vi "APU + Event Timing v6 single shot.vi"() -> ()   [LabVIEW 2013]
uses:
  IP Source/APU/Input.ctl
  IP Source/APU/Output.ctl
  IP Source/APU/Settings.ctl
  IP Source/ECU Event/Timing/Capture Output.ctl
  IP Source/ECU Event/Timing/Measure Settings.ctl
  IP Source/Version Token.ctl
  IP Source/ECU Event/Timing/Measure Output.ctl
  IP Source/APU/Shared Settings.ctl
  <vilib>/Platform/TimedLoop/XDataNode/timing_clust.ctl
  <vilib>/Platform/TimedLoop/XDataNode/nitl_modes.ctl
  <vilib>/Platform/TimedLoop/XDataNode/wakeup.ctl
  IP Source/ECU Event/Timing/Capture Settings.ctl
  <vilib>/rvi/Emulation/niFpgaSctlEmulationGetInTimedLoop.vi
  <vilib>/rvi/Emulation/niFpgaEmulationReportErrorSimple.vi
  <vilib>/rvi/Emulation/niFpgaGetClockAttributes.vi
  <vilib>/rvi/Emulation/niFpgaCriticalErrorInLSC.vi
  IP Source/ECU Event/Timing/Measure Events (40MHz).vi
  <vilib>/rvi/eio/common/nirviEmuTemplateMethod_errors.vi
  <vilib>/Platform/TimedLoop/XDataNode/XDataNode.xnode
  <vilib>/eio/EIONode/EIONode.xnode
  <vilib>/Platform/TimedLoop/XDataNode/XDNodeRunTimeDep.lvlib
  IP Source/ECU Event/Timing/ECU Event Timing.lvlib
  IP Source/APU/APU.lvlib
  IP Source/Engine Simulation Toolkit.lvlib
panel:
  in  "shared settings.my apu":T1 {"cycle start" format="%#.15g"}
  in  "go.my apu":bool
  out "measure output.fi 6":T2
  out "measure output.fi 5":T2
  out "measure output.fi 4":T2
  out "measure output.fi 3":T2
  out "measure output.fi 2":T2
  out "measure output.fi 1":T2
  out "measure output.spark 6":T2
  out "measure output.spark 5":T2
  out "measure output.spark 4":T2
  out "measure output.spark 3":T2
  out "measure output.spark 2":T2
  out "measure output.spark 1":T2
  in  "est.version":T3
  out "Output.fi 1 shot 1":T4
  out "Output.fi 2 shot 1":T4
  out "Output.fi 3 shot 1":T4
  out "Output.fi 4 shot 1":T4
  out "Output.fi 5 shot 1":T4
  out "Output.fi 6 shot 1":T4
  in  "Settings.fi 1":T5
  in  "Settings.fi 2":T5
  in  "Settings.fi 3":T5
  in  "Settings.fi 4":T5
  in  "Settings.fi 5":T5
  in  "Settings.fi 6":T5
  in  "Settings.spark 6":T5
  in  "Settings.spark 5":T5
  in  "Settings.spark 4":T5
  in  "Settings.spark 3":T5
  in  "Settings.spark 2":T5
  in  "Settings.spark 1":T5
  out "Output.spark 1 shot 1":T4
  out "Output.spark 2 shot 1":T4
  out "Output.spark 3 shot 1":T4
  out "Output.spark 4 shot 1":T4
  out "Output.spark 5 shot 1":T4
  out "Output.spark 6 shot 1":T4
  in  "Settings.my apu":T6 caption="settings"
  out "Output.my apu":T7 caption="output"
  in  "Input.my apu":T8={"desired speed"=0.0, "reset"=TRUE} caption="input"
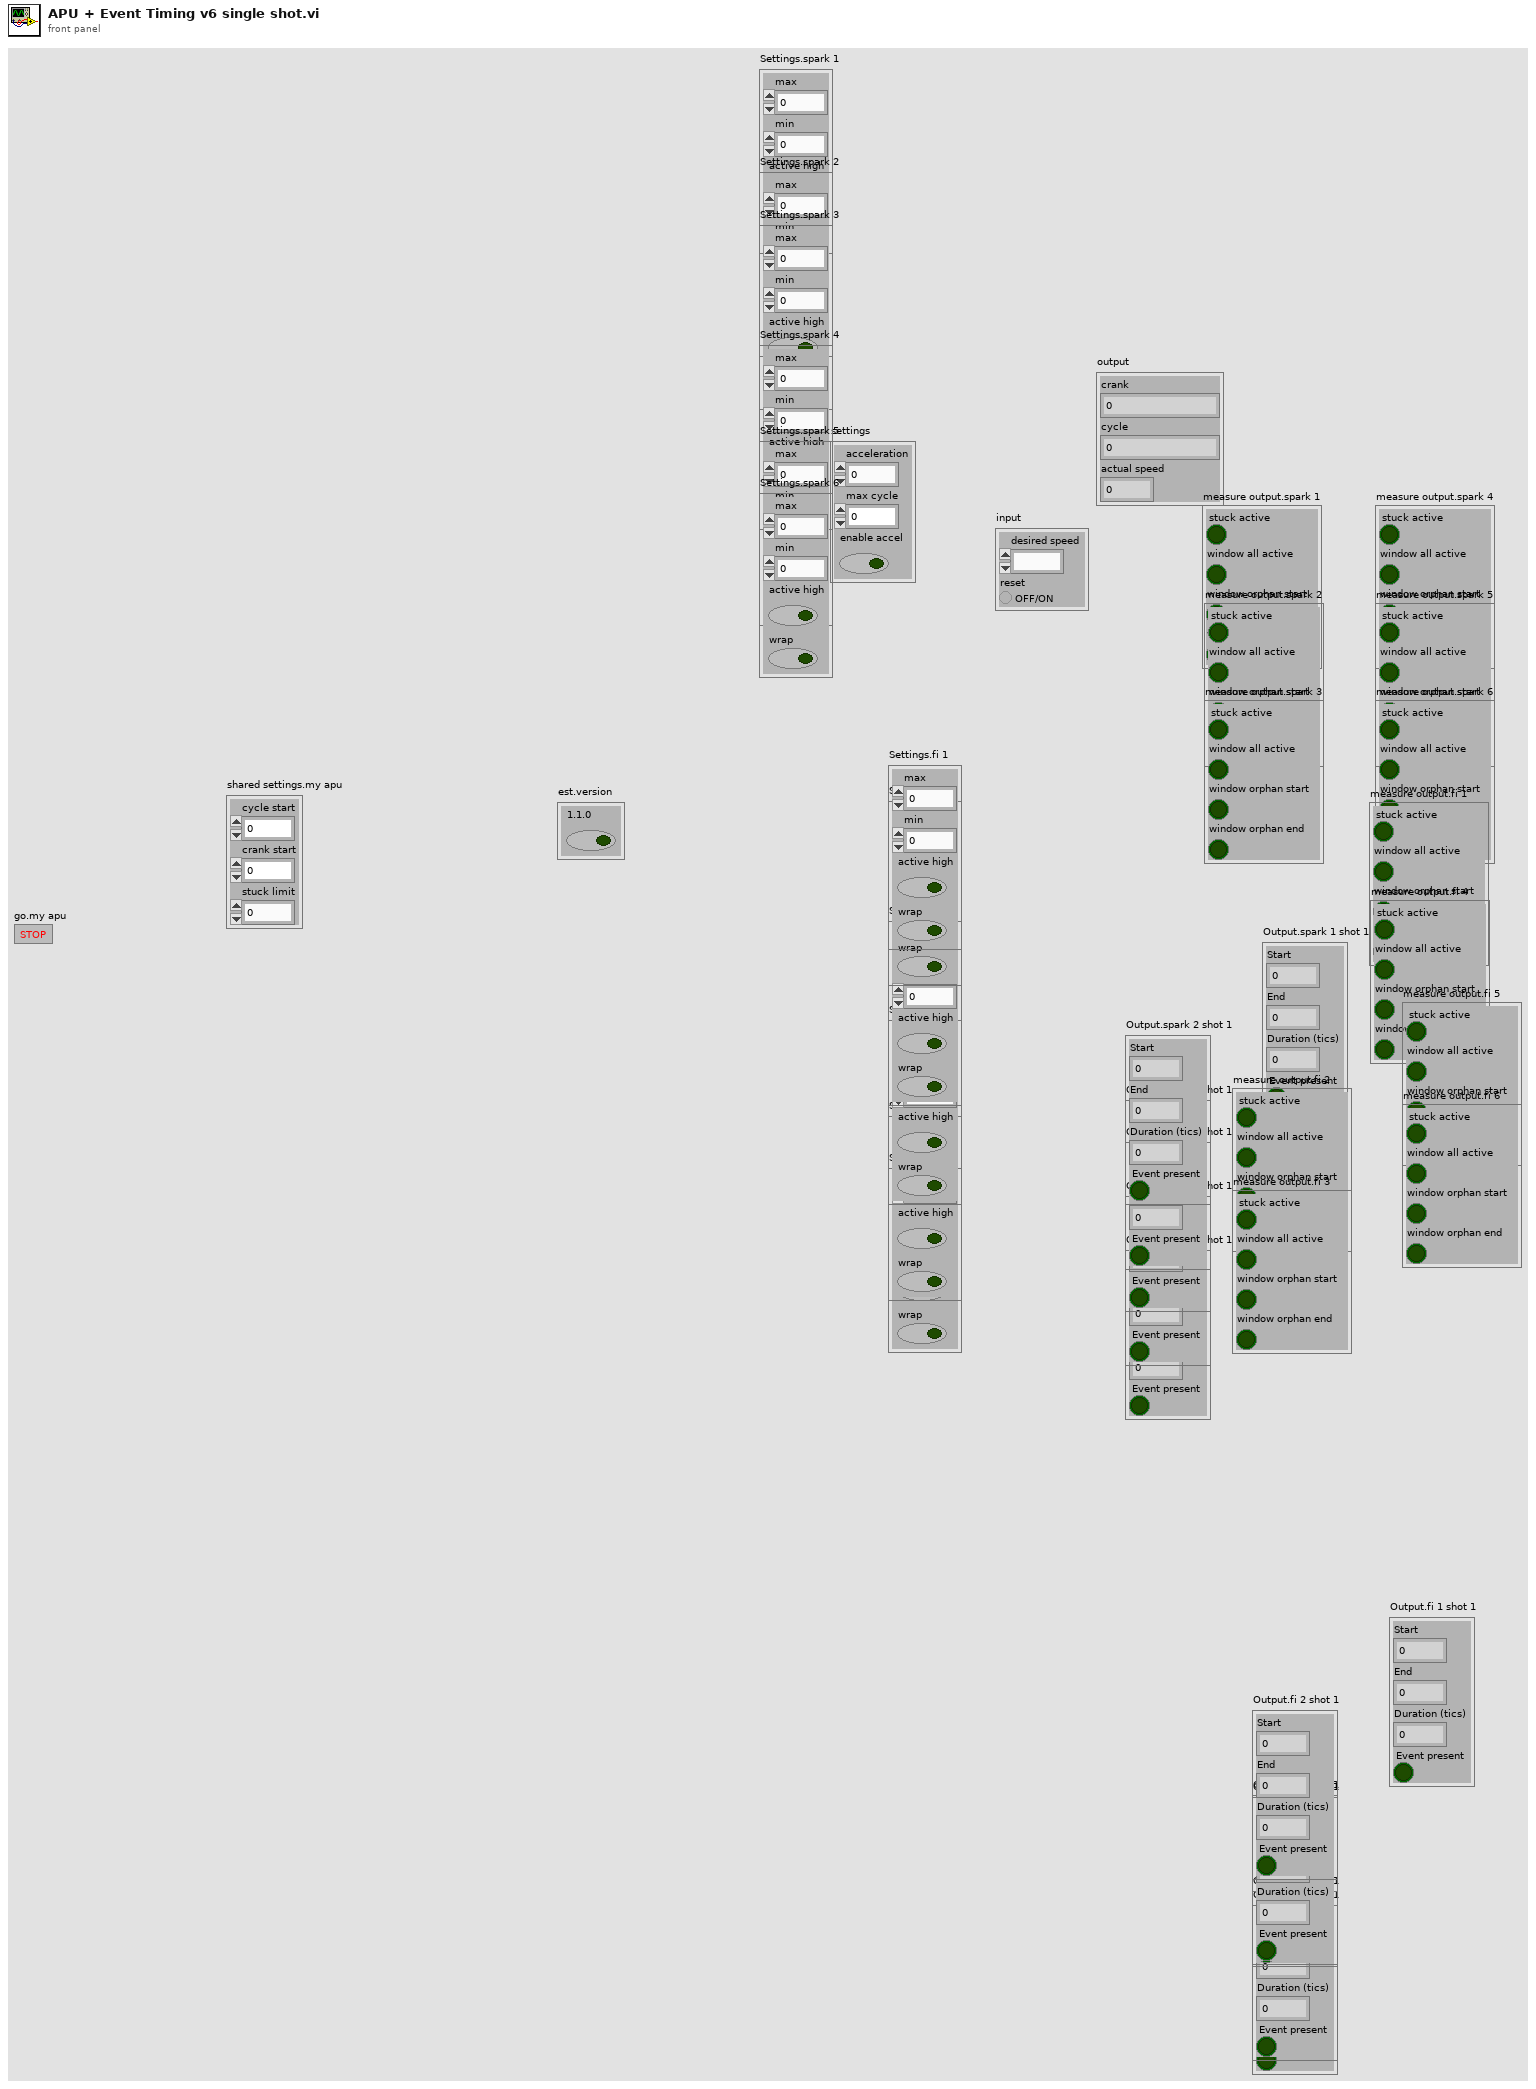
[diagram p1: front panel]
types:
  T1 = typedef "Engine Simulation Toolkit.lvlib/APU.lvlib/Shared Settings.ctl" = cluster{"cycle start":fxp<+,2,2>, "crank start":u16, "stuck limit":fxp<+,18,18>}
  T2 = typedef "Engine Simulation Toolkit.lvlib/ECU Event Timing.lvlib/Measure Output.ctl" = cluster{"stuck active":bool, "window all active":bool, "window orphan start":bool, "window orphan end":bool}
  T3 = typedef "Engine Simulation Toolkit.lvlib/Version Token.ctl" = cluster{"1.1.0":bool}
  T4 = typedef "Engine Simulation Toolkit.lvlib/ECU Event Timing.lvlib/Capture Output.ctl" = cluster{"Start":u16, "End":u16, "Duration (tics)":fxp<+,18,18>, "Event present":bool}
  T5 = typedef "Engine Simulation Toolkit.lvlib/ECU Event Timing.lvlib/Measure Settings.ctl" = cluster{"max":u16, "min":u16, "active high":bool, "wrap":bool}
  T6 = typedef "Engine Simulation Toolkit.lvlib/APU.lvlib/Settings.ctl" = cluster{"acceleration":fxp<+,18,-20>, "max cycle":fxp<+,2,2>, "enable accel":bool}
  T7 = typedef "Engine Simulation Toolkit.lvlib/APU.lvlib/Output.ctl" = cluster{"crank":u16, "cycle":u16, "actual speed":fxp<+/-,23,2>}
  T8 = typedef "Engine Simulation Toolkit.lvlib/APU.lvlib/Input.ctl" = cluster{"desired speed":fxp<+/-,23,2>, "reset":bool}
  T9 = typedef "XDNodeRunTimeDep.lvlib/timing_clust.ctl" = cluster{"Expected End [f-1]":u64, "Actual End [f-1]":u64, "Finished Late? [f-1]":bool, "Expected End [i-1]":u64, "Actual End [i-1]":u64, "Finished Late? [i-1]":bool, "Expected Start [i]":u64, "Actual Start [i]":u64, "Expected Start [f]":u64, "Actual Start [f]":u64, "Source Name":string, "Structure Name":string, "Period":i64, "Deadline":i64, "Offset":i64, "Start":i64, "Priority":i32, "Timeout":i32, "Mode":T10, "Wakeup Reason":T11, "Error":errorcluster, "Source Type":string, "Secondary Source Type":string, "Global End Time":u64, "Global Start Time":u64, "Frame Duration":u64, "Iteration Duration":u64, "Assigned CPU":i32, "I/O Scan Engine Mode":u32}
  T10 = typedef "XDNodeRunTimeDep.lvlib/nitl_modes.ctl" = enum32{"No Change", "Process missed periods, maintain original phase", "Discard missed periods, maintain original phase", "Process missed periods, ignore original phase", "Discard missed periods, ignore original phase"}
  T11 = typedef "XDNodeRunTimeDep.lvlib/wakeup.ctl" = enum32{"Normal", "Aborted", "Asynchronous wakeup", "Timing source error", "Timed loop error", "Timeout"}
  T12 = typedef "Engine Simulation Toolkit.lvlib/APU.lvlib/Register Bus.ctl" = cluster{"Speed":refnum<k21>, "Crank Angle":refnum<k21>, "Cycle Angle":refnum<k21>, "Crank Count":refnum<k21>, "Cycle Count":refnum<k21>, "1.25 MHz Counter":refnum<k21>, "shared settings":T1}
  T13 = typedef "Engine Simulation Toolkit.lvlib/ECU Event Timing.lvlib/Capture Settings.ctl" = u8
  T14 = typedef "Engine Simulation Toolkit.lvlib/ECU Event Timing.lvlib/Measured Data.ctl" = cluster{"start":u16, "end":u16, "duration (tics)":fxp<+,18,18>, "window end":bool, "window begin":bool, "pulse end":bool, "pulse #":u8}
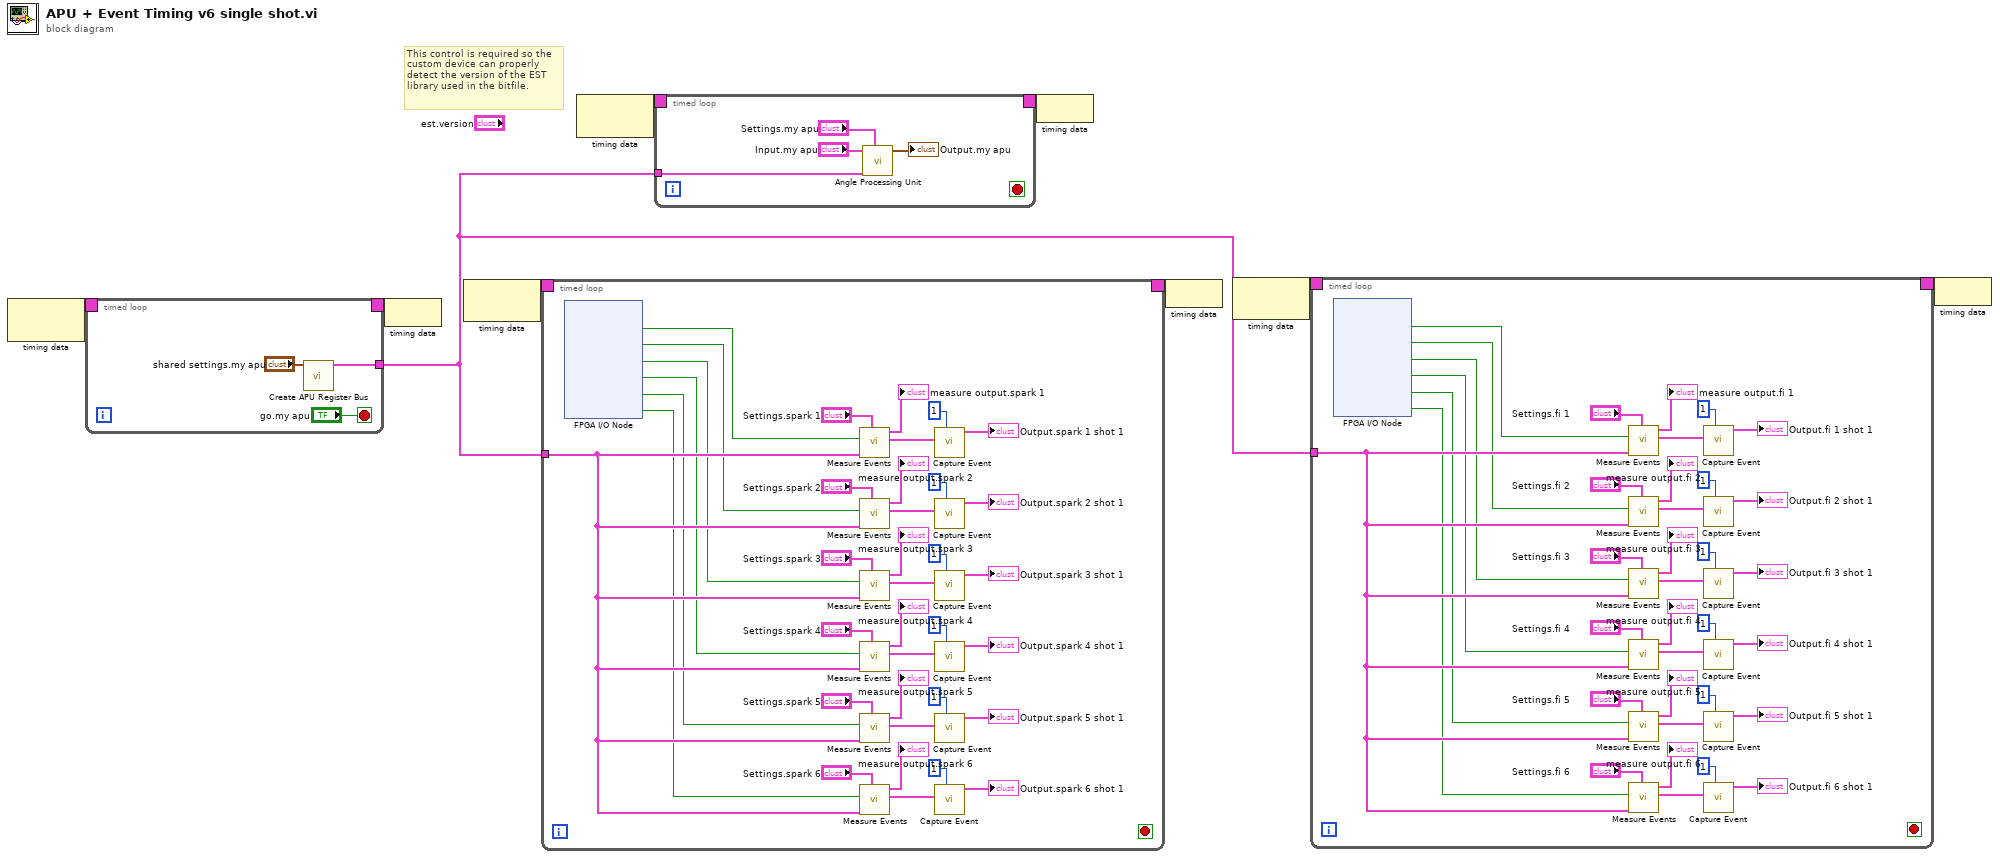
[diagram p0: block diagram]
diagram:
  # "This control is required so the custom device can properly detect the version of the EST library used in the bitfile."
  n1 = node-c288() -> (w3:T9)  [unwired: 1 in]
  n2 = timed-loop {
    timing: w3 -> [_]
    timing-out: [_] -> w2
    tunnel: [w12] -> w1
    stop <- "go.my apu" stop-if-true
    n3 = call "Create APU Register Bus.vi"("shared settings.<user name>"="shared settings.my apu") -> ("register bus"=w12:T12)  [unwired: 10 in]
  }
  n4 = node-c288(w2) -> ()
  n5 = node-c288() -> (w7:T9)  [unwired: 1 in]
  n6 = timed-loop {
    timing: w7 -> [_]
    timing-out: [_] -> w6
    tunnel: w1 -> [w45]
    stop <- _ stop-if-true
    n7 = xnode "FPGA I/O Node"() -> ("DIO0_1"=w26:bool, "DIO1_1"=w25:bool, "DIO2_1"=w24:bool, "DIO3_1"=w23:bool, "DIO4_1"=w22:bool, "DIO5_1"=w21:bool)  [unwired: 6 in, 6 out]
    n8 = call-poly "Measure Events.vi"("settings.<user name>"="Settings.spark 1", "register bus"=w45, "event"=w26) -> ("measured data"=w44:T14, "status.<user name>"=→"measure output.spark 1":T2)  [unwired: 7 in]
    n9 = call-poly "Measure Events.vi"("settings.<user name>"="Settings.spark 2", "register bus"=w45, "event"=w25) -> ("measured data"=w37:T14, "status.<user name>"=→"measure output.spark 2":T2)  [unwired: 7 in]
    n10 = call-poly "Measure Events.vi"("settings.<user name>"="Settings.spark 3", "register bus"=w45, "event"=w24) -> ("measured data"=w36:T14, "status.<user name>"=→"measure output.spark 3":T2)  [unwired: 7 in]
    n11 = call-poly "Measure Events.vi"("settings.<user name>"="Settings.spark 4", "register bus"=w45, "event"=w23) -> ("measured data"=w35:T14, "status.<user name>"=→"measure output.spark 4":T2)  [unwired: 7 in]
    n12 = call-poly "Measure Events.vi"("settings.<user name>"="Settings.spark 5", "register bus"=w45, "event"=w22) -> ("measured data"=w34:T14, "status.<user name>"=→"measure output.spark 5":T2)  [unwired: 7 in]
    n13 = call-poly "Measure Events.vi"("settings.<user name>"="Settings.spark 6", "register bus"=w45, "event"=w21) -> ("measured data"=w33:T14, "status.<user name>"=→"measure output.spark 6":T2)  [unwired: 7 in]
    n14 = call "Capture Event.vi"("event # to capture"=T13 1 ("Settings.spark 1 shot 1"), "measured data"=w44) -> ("capture.<user name>"=→"Output.spark 1 shot 1":T4)  [unwired: 9 in]
    n15 = call "Capture Event.vi"("event # to capture"=T13 1 ("Settings.spark 2 shot 1"), "measured data"=w37) -> ("capture.<user name>"=→"Output.spark 2 shot 1":T4)  [unwired: 9 in]
    n16 = call "Capture Event.vi"("event # to capture"=T13 1 ("Settings.spark 3 shot 1"), "measured data"=w36) -> ("capture.<user name>"=→"Output.spark 3 shot 1":T4)  [unwired: 9 in]
    n17 = call "Capture Event.vi"("event # to capture"=T13 1 ("Settings.spark 4 shot 1"), "measured data"=w35) -> ("capture.<user name>"=→"Output.spark 4 shot 1":T4)  [unwired: 9 in]
    n18 = call "Capture Event.vi"("event # to capture"=T13 1 ("Settings.spark 5 shot 1"), "measured data"=w34) -> ("capture.<user name>"=→"Output.spark 5 shot 1":T4)  [unwired: 9 in]
    n19 = call "Capture Event.vi"("event # to capture"=T13 1 ("Settings.spark 6 shot 1"), "measured data"=w33) -> ("capture.<user name>"=→"Output.spark 6 shot 1":T4)  [unwired: 9 in]
  }
  n20 = node-c288() -> (w9:T9)  [unwired: 1 in]
  n21 = timed-loop {
    timing: w9 -> [_]
    timing-out: [_] -> w8
    tunnel: w1 -> [w54]
    stop <- _ stop-if-true
    n22 = call "Angle Processing Unit.vi"("settings.<user name>"="Settings.my apu", "register bus"=w54, "input.<user name>"="Input.my apu") -> ("output.<user name>"=→"Output.my apu":T7)  [unwired: 8 in]
  }
  n23 = node-c288(w8) -> ()
  n24 = node-c288(w6) -> ()
  n25 = node-c288() -> (w5:T9)  [unwired: 1 in]
  n26 = timed-loop {
    timing: w5 -> [_]
    timing-out: [_] -> w4
    tunnel: w1 -> [w90]
    stop <- _ stop-if-true
    n27 = xnode "FPGA I/O Node"() -> ("DIO0_0"=w71:bool, "DIO1_0"=w70:bool, "DIO2_0"=w69:bool, "DIO3_0"=w68:bool, "DIO4_0"=w67:bool, "DIO5_0"=w66:bool)  [unwired: 6 in, 6 out]
    n28 = call-poly "Measure Events.vi"("settings.<user name>"="Settings.fi 1", "register bus"=w90, "event"=w71) -> ("measured data"=w89:T14, "status.<user name>"=→"measure output.fi 1":T2)  [unwired: 7 in]
    n29 = call-poly "Measure Events.vi"("settings.<user name>"="Settings.fi 2", "register bus"=w90, "event"=w70) -> ("measured data"=w82:T14, "status.<user name>"=→"measure output.fi 2":T2)  [unwired: 7 in]
    n30 = call-poly "Measure Events.vi"("settings.<user name>"="Settings.fi 3", "register bus"=w90, "event"=w69) -> ("measured data"=w81:T14, "status.<user name>"=→"measure output.fi 3":T2)  [unwired: 7 in]
    n31 = call-poly "Measure Events.vi"("settings.<user name>"="Settings.fi 4", "register bus"=w90, "event"=w68) -> ("measured data"=w80:T14, "status.<user name>"=→"measure output.fi 4":T2)  [unwired: 7 in]
    n32 = call-poly "Measure Events.vi"("settings.<user name>"="Settings.fi 5", "register bus"=w90, "event"=w67) -> ("measured data"=w79:T14, "status.<user name>"=→"measure output.fi 5":T2)  [unwired: 7 in]
    n33 = call-poly "Measure Events.vi"("settings.<user name>"="Settings.fi 6", "register bus"=w90, "event"=w66) -> ("measured data"=w78:T14, "status.<user name>"=→"measure output.fi 6":T2)  [unwired: 7 in]
    n34 = call "Capture Event.vi"("event # to capture"=T13 1 ("Settings.fi 1 shot 1"), "measured data"=w89) -> ("capture.<user name>"=→"Output.fi 1 shot 1":T4)  [unwired: 9 in]
    n35 = call "Capture Event.vi"("event # to capture"=T13 1 ("Settings.fi 2 shot 1"), "measured data"=w82) -> ("capture.<user name>"=→"Output.fi 2 shot 1":T4)  [unwired: 9 in]
    n36 = call "Capture Event.vi"("event # to capture"=T13 1 ("Settings.fi 3 shot 1"), "measured data"=w81) -> ("capture.<user name>"=→"Output.fi 3 shot 1":T4)  [unwired: 9 in]
    n37 = call "Capture Event.vi"("event # to capture"=T13 1 ("Settings.fi 4 shot 1"), "measured data"=w80) -> ("capture.<user name>"=→"Output.fi 4 shot 1":T4)  [unwired: 9 in]
    n38 = call "Capture Event.vi"("event # to capture"=T13 1 ("Settings.fi 5 shot 1"), "measured data"=w79) -> ("capture.<user name>"=→"Output.fi 5 shot 1":T4)  [unwired: 9 in]
    n39 = call "Capture Event.vi"("event # to capture"=T13 1 ("Settings.fi 6 shot 1"), "measured data"=w78) -> ("capture.<user name>"=→"Output.fi 6 shot 1":T4)  [unwired: 9 in]
  }
  n40 = node-c288(w4) -> ()
